vi "Add Port.vi"(8 "error in":errorcluster, 10 "port number":u16, 11 "custom device ref":T1 format="%.0x") -> (0 "error out":errorcluster, 2 "port":T1 format="%.0x", 3 "custom device ref out":T1 format="%.0x")   [LabVIEW 2020, in "AIM MIL-STD-1553 Scripting.lvlib"]
doc: "Adds the specified <b>port</b> (number) to the custom device system definition and returns the newly added <b>port</b> reference."
uses:
  AIM MIL-STD-1553 Scripting.lvlib
  <vilib>/NI VeriStand/Custom Device API/Custom Device API.lvlib
  Constants.vi
  <vilib>/NI VeriStand/Custom Device API/Custom Device Item Ref.ctl
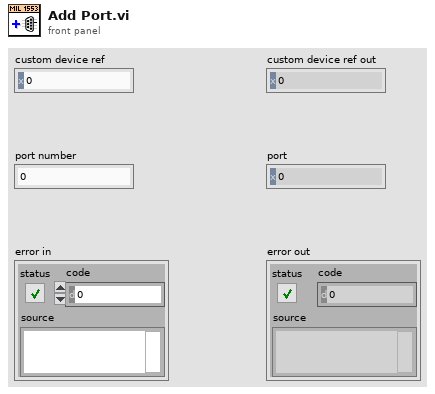
[diagram p1: front panel]
types:
  T1 = typedef "Custom Device API.lvlib/Custom Device Item Ref.ctl" = u64
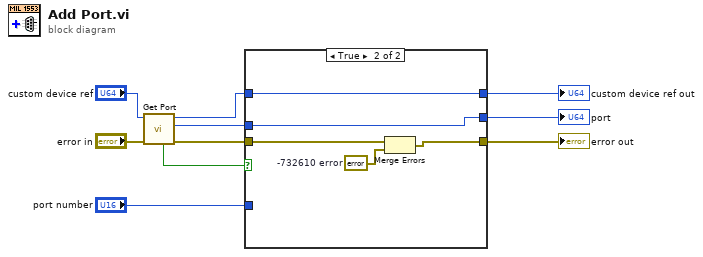
[diagram p0: block diagram]
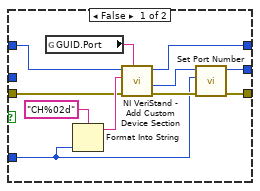
[diagram p2: hidden frame]
diagram:
  n1 = call "Get Port.vi"("error in"="error in", "custom device ref"="custom device ref") -> ("error out"=w2:errorcluster, "port"=w3:T1, "custom device ref out"=w4:T1, "found"=w1:bool)  [unwired: 6 in]
  n2 = case shown="True" w1 {
    tunnel: [w19 w26] -> w10
    tunnel: [w16 w24] -> w9
    tunnel: "port number" -> [w15 _]
    tunnel: [w14 w25] -> w7
    tunnel: w2 -> [w12 w23]
    tunnel: w4 -> [w11 w26]
    tunnel: w3 -> [_ w25]
    frame False {
      n3 = global read "Constants.vi" "GUID.Port"() -> (w13:string)
      n4 = Format Into String(format string="CH%02d", w15) -> (resulting string=w20:string)  [unwired: 2 in, 1 out]
      n5 = call <vilib>:"NI VeriStand - Add Custom Device Section.vi"("GUID (Default Section)"=w13, "error in (no error)"=w12, "Section Name"=w20, "Parent Ref in"=w11) -> ("error out"=w17:errorcluster, "Section Ptr"=w18:T1, "Parent Ref out"=w19:T1)  [unwired: 4 in, 1 out]
      n6 = call "Set Port Number.vi"("error in"=w17, "port number"=w15, "port in"=w18) -> ("error out"=w16:errorcluster, "port out"=w14:T1)  [unwired: 7 in]
    }
    frame True {
      w22 = errorcluster {"status"=TRUE, "code"=-732610, "source"="Tried to add a hardware channel to this BIU when one already exists.  The AIM MIL-STD 1553 custom device only supports one hardware channel in the parameters file."}  # -732610 error
      n7 = Merge Errors(w23, w22) -> (w24:errorcluster)
    }
  }
  "custom device ref out" <- w10
  "error out" <- w9
  "port" <- w7
